vi "Drive_setAbortPositionControl.vi"(8 "error in (no error)":errorcluster, 10 "Abort? (F)":bool) -> (0 "error out":errorcluster)   [LabVIEW 2009, in "Drive.lvlib"]
uses:
  Drive.lvlib
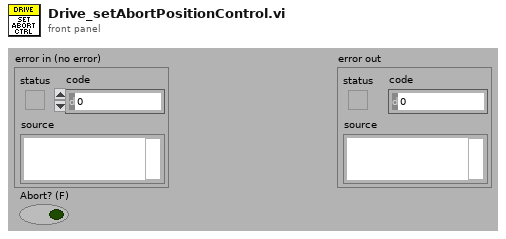
[diagram p1: front panel]
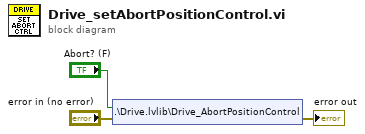
[diagram p0: block diagram]
diagram:
  n1 = shared-variable ".\\Drive.lvlib\\Drive_AbortPositionControl"("Abort? (F)", error in="error in (no error)") -> (error out=→"error out":errorcluster)
